vi "Read Signal Generator.lvclass.vi"(11 "AM-AM in":refnum<class "AM-AM.lvclass">) -> (2 "Signal Generator.lvclass":refnum<class "Signal Generator.lvclass">, 3 "AM-AM out":refnum<class "AM-AM.lvclass">)   [LabVIEW 2020, in "AM-AM.lvclass"]
uses:
  AM-AM.lvclass
  Instruments/Signal Generator/Signal Generator.lvclass
  AM-AM.lvclass/AM-AM.ctl
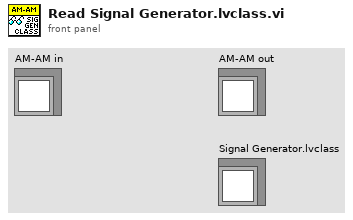
[diagram p1: front panel]
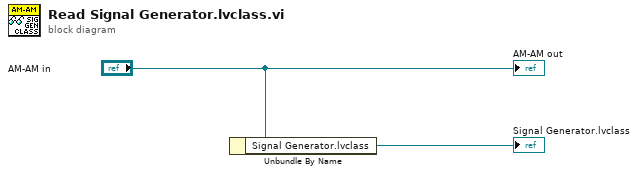
[diagram p0: block diagram]
diagram:
  n1 = Unbundle By Name("AM-AM in") -> ("Signal Generator.lvclass"=→"Signal Generator.lvclass":refnum<class "Signal Generator.lvclass">)
  "AM-AM out" <- "AM-AM in"
